vi "Do.vi"(8 "error in (no error)":errorcluster, 10 "Actor in":refnum<class "Actor.lvclass">, 11 "Update from Process Msg":refnum<class "Update from Process Msg.lvclass">) -> (0 "error out":errorcluster, 2 "Actor out":refnum<class "Actor.lvclass">)   [LabVIEW 2014, in "States.lvlib" / "Update from Process Msg.lvclass"]
doc: "This VI delivers the message to the actor by calling the appropriate method(s) on the actor."
uses:
  Update from Process Msg.lvclass
  <vilib>/ActorFramework/Actor/Actor.lvclass
  Process State/CoordinatorState.lvclass
  Update from Process Msg.lvclass/Update from Process Msg.ctl
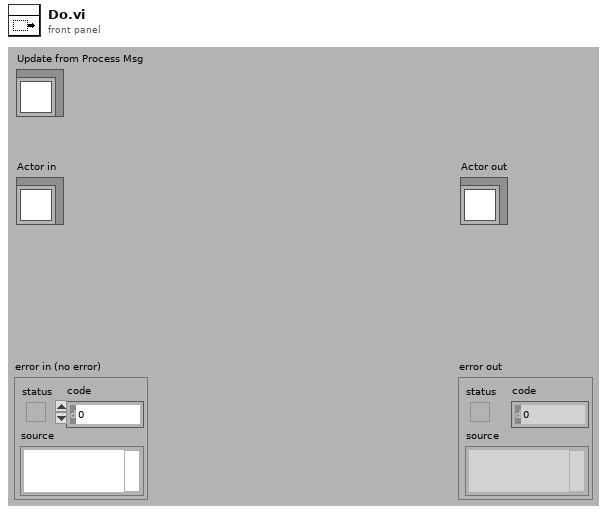
[diagram p1: front panel]
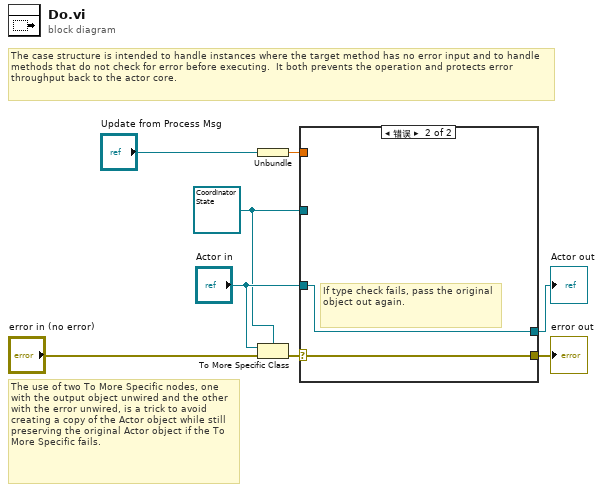
[diagram p0: block diagram]
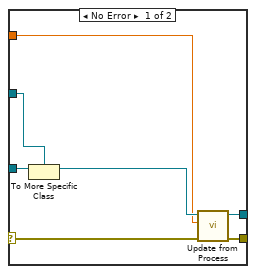
[diagram p2: hidden frame]
diagram:
  w1 = refnum<class "CoordinatorState.lvclass"> refnum ("Process States.lvlib:Process State.lvclass")
  # "The use of two To More Specific nodes, one with the output object unwired and the other with the error unwired, is a trick to avoid creating a copy of the Actor object while still preserving the original Actor object if the To More Specific fails."
  # "The case structure is intended to handle instances where the target method has no error input and to handle methods that do not check for error before executing.  It both prevents the operation and protects error throughput back to the actor core."
  n1 = Unbundle("Update from Process Msg") -> (w3:dbl)
  n2 = To More Specific Class(target class=w1, reference="Actor in", error in="error in (no error)") -> (error out=w7:errorcluster)  [unwired: 1 out]
  n3 = case shown="错误" w7 {
    selector: w7 -> [w13 w16]
    tunnel: [w15 w16] -> w6
    tunnel: [w14 w17] -> w5
    tunnel: "Actor in" -> [w12 w17]
    tunnel: w1 -> [w11 _]
    tunnel: w3 -> [w9 _]
    frame No Error {
      n4 = To More Specific Class(target class=w11, reference=w12) -> (specific class reference=w10:refnum<class "CoordinatorState.lvclass">)  [unwired: 1 in, 1 out]
      n5 = call-dynamic "Update from Process.vi"("error in (no error)"=w13, "Value"=w9, "Process State in"=w10) -> ("error out"=w15:errorcluster, "Process State out"=w14:refnum<class "State Actor.lvclass">)  [unwired: 7 in]
    }
    frame Error {
      # "If type check fails, pass the original object out again."
    }
  }
  "error out" <- w6
  "Actor out" <- w5
